vi "Calculator-setup.vi"(11 "test case ID":string) -> (0 "error out":errorcluster={"status"=TRUE, "code"=0, "source"=""}, 1 "Operation":T1, 2 "b":dbl, 3 "a":dbl)   [LabVIEW 2018]
doc: "The setup VI should be executed before the VI under test in the harness VI. In this VI you can prepare the environment and the inputs of the VI under test.\n\nSee the Help Document for more information. (<b>Help</b> > <b>IncQuery Labs</b> > <b>InstaCoverage</b> > <b>InstaCoverage Help...</b>)"
uses:
  Control 1.ctl
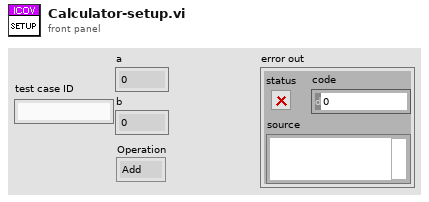
[diagram p1: front panel]
types:
  T1 = typedef "Control 1.ctl" = enum16{"Add", "Subtract", "Multiply", "Divide"}
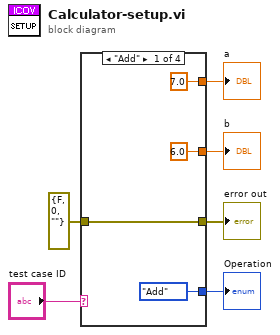
[diagram p0: block diagram]
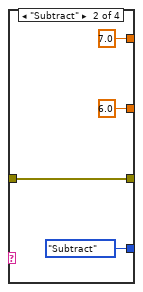
[diagram p2: hidden frame]
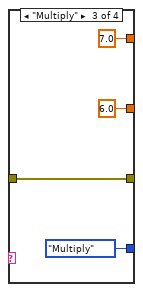
[diagram p3: hidden frame]
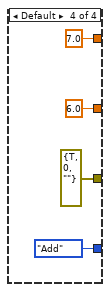
[diagram p4: hidden frame]
diagram:
  n1 = case shown="\"Add\"" "test case ID" {
    tunnel: [7.0 ("a") 7.0 ("a") 7.0 ("a") 7.0 ("a")] -> w5
    tunnel: [6.0 ("b") 6.0 ("b") 6.0 ("b") 6.0 ("b")] -> w4
    tunnel: [Control_1."Add" ("Operation") Control_1."Subtract" ("Operation") Control_1."Multiply" ("Operation") Control_1."Add" ("Operation")] -> w3
    tunnel: [w7 w11 w15 errorcluster {"status"=TRUE, "code"=0, "source"=""} ("error in (no error)")] -> w2
    tunnel: errorcluster {"status"=FALSE, "code"=0, "source"=""} ("error in (no error)") -> [w7 w11 w15 _]
    frame "Add" {
    }
    frame "Subtract" {
    }
    frame "Multiply" {
    }
    frame Default {
    }
  }
  "a" <- w5
  "b" <- w4
  "Operation" <- w3
  "error out" <- w2
